vi "Scale.vi"(8 "error in (no error)":errorcluster, 10 "Scale Factor":dbl, 11 "Text in":refnum<class "Text.lvclass">) -> (0 "error out":errorcluster, 3 "Text out":refnum<class "Text.lvclass">)   [LabVIEW 2021, in "Picture2D.lvlib" / "Text.lvclass"]
uses:
  Text.lvclass
  Text.lvclass/Text.ctl
  Shape/Shape.lvclass
  Font/Font.lvclass
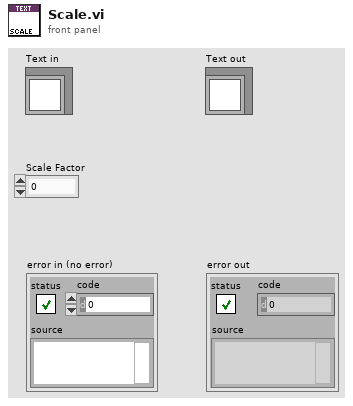
[diagram p1: front panel]
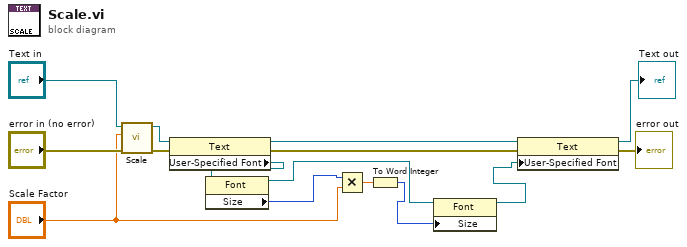
[diagram p0: block diagram]
diagram:
  n1 = call-parent "Scale.vi"("error in (no error)"="error in (no error)", "Scale Factor"="Scale Factor", "Shape in"="Text in") -> ("error out"=w7:errorcluster, "Shape out"=w13:refnum<class "Text.lvclass">)  [unwired: 7 in]
  n2 = property class="Text"(reference=w13, error in=w7) -> (reference out=w11:refnum<class "Text.lvclass">, error out=w8:errorcluster, "User-Specified Font"=w5:refnum<class "Font.lvclass">)
  n3 = property class="Font"(reference=w5) -> (reference out=w1:refnum<class "Font.lvclass">, "Size"=w4:i16)  [unwired: 1 in, 1 out]
  n4 = Multiply(x=w4, y="Scale Factor") -> (x*y=w9:dbl)
  n5 = To Word Integer(number=w9) -> (16bit integer=w3:i16)
  n6 = property class="Font"(reference=w1, "Size"=w3) -> (reference out=w2:refnum<class "Font.lvclass">)  [unwired: 1 in, 1 out]
  n7 = property class="Text"(reference=w11, error in=w8, "User-Specified Font"=w2) -> (reference out=→"Text out":refnum<class "Text.lvclass">, error out=→"error out":errorcluster)
